vi "Set Frequency.vi"(8 "error in (no error)":errorcluster, 10 "Frequency (1000Hz)":dbl=1000.0, 11 "PWM in":refnum<class "LINX-PCA9865 PWM.lvclass">) -> (0 "error out":errorcluster, 3 "PWM out":refnum<class "LINX-PCA9865 PWM.lvclass">)   [LabVIEW 2019, in "LINX-PCA9865 PWM.lvclass"]
uses:
  LINX-PCA9865 PWM.lvclass
panel:
  out "Prescale Value":dbl
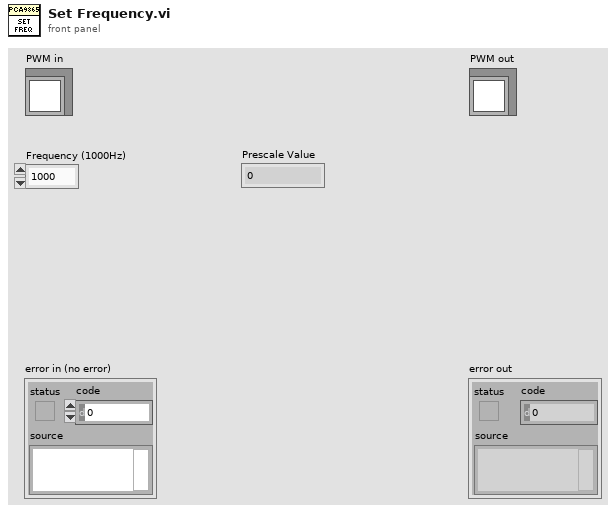
[diagram p1: front panel]
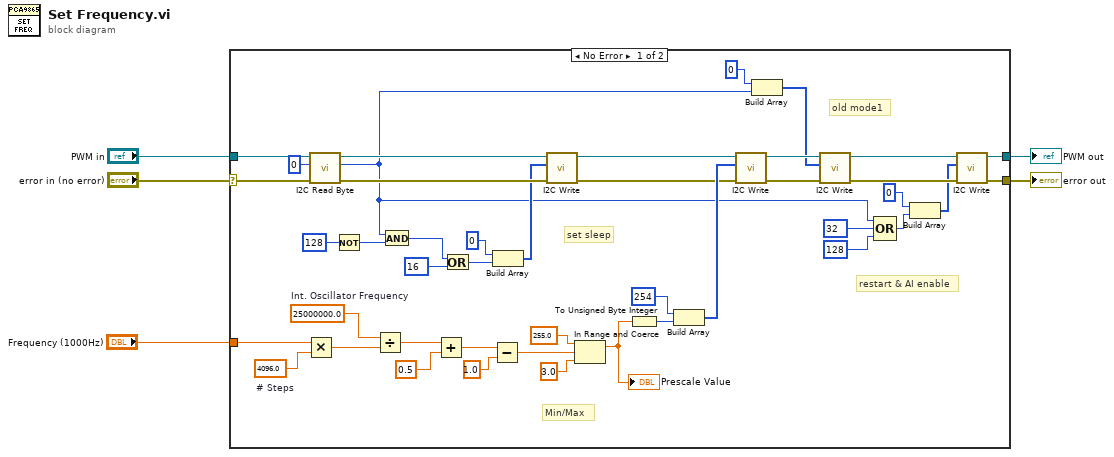
[diagram p0: block diagram]
diagram:
  n1 = case shown="No Error" "error in (no error)" {
    selector: "error in (no error)" -> [w32 w50]
    tunnel: [w13 w50] -> w4
    tunnel: [w12 w49] -> w2
    tunnel: "PWM in" -> [w33 w49]
    tunnel: "Frequency (1000Hz)" -> [w48 _]
    frame No Error {
      w47 = 4096.0  # # Steps
      w46 = 25000000.0  # Int. Oscillator Frequency
      # "set sleep"
      # "old mode1"
      # "restart & AI enable"
      # "Min/Max"
      n2 = Multiply(x=w48, y=w47) -> (x*y=w45:dbl)
      n3 = call "I2C Read Byte.vi"("error in (no error)"=w32, "Address"=u8 0, "LINX-PCA9865 PWM in"=w33) -> ("error out"=w26:errorcluster, "Byte Read"=w11:u8, "LINX-PCA9865 PWM out"=w23:refnum<class "LINX-PCA9865 PWM.lvclass">)  [unwired: 6 in]
      n4 = Not(x=u8 128) -> (.not. x?=w29:u8)
      n5 = Divide(x=w46, y=w45) -> (x/y=w44:dbl)
      n6 = And(x=w11, y=w29) -> (x .and. y?=w28:u8)
      n7 = Add(x=w44, y=0.5 ("x")) -> (x+y=w42:dbl)
      n8 = Or(x=w28, y=u8 16) -> (x .or. y?=w21:u8)
      n9 = Subtract(x=w42, y=1.0) -> (x-y=w40:dbl)
      n10 = Build Array(u8 0 ("Address"), w21) -> (w20:u8[])
      n11 = call "I2C Write.vi"("error in (no error)"=w26, "Bytes to Write"=w20, "LINX-PCA9865 PWM in"=w23) -> ("error out"=w25:errorcluster, "LINX-PCA9865 PWM out"=w24:refnum<class "LINX-PCA9865 PWM.lvclass">)  [unwired: 7 in]
      n12 = In Range and Coerce(upper limit=255.0, x=w40, lower limit=3.0) -> (coerced(x)=w37:dbl)  [unwired: 1 out]
      "Prescale Value" <- w37
      n13 = To Unsigned Byte Integer(number=w37) -> (unsigned 8bit integer=w36:u8)
      n14 = Build Array(u8 254 ("unsigned 8bit integer"), w36) -> (w35:u8[])
      n15 = call "I2C Write.vi"("error in (no error)"=w25, "Bytes to Write"=w35, "LINX-PCA9865 PWM in"=w24) -> ("error out"=w19:errorcluster, "LINX-PCA9865 PWM out"=w18:refnum<class "LINX-PCA9865 PWM.lvclass">)  [unwired: 7 in]
      n16 = Build Array(u8 0 ("Address"), w11) -> (w16:u8[])
      n17 = call "I2C Write.vi"("error in (no error)"=w19, "Bytes to Write"=w16, "LINX-PCA9865 PWM in"=w18) -> ("error out"=w14:errorcluster, "LINX-PCA9865 PWM out"=w15:refnum<class "LINX-PCA9865 PWM.lvclass">)  [unwired: 7 in]
      n18 = Compound Arithmetic op=OR(w11, u8 32, u8 128) -> (w7:u8)
      n19 = Build Array(u8 0 ("Address"), w7) -> (w6:u8[])
      n20 = call "I2C Write.vi"("error in (no error)"=w14, "Bytes to Write"=w6, "LINX-PCA9865 PWM in"=w15) -> ("error out"=w13:errorcluster, "LINX-PCA9865 PWM out"=w12:refnum<class "LINX-PCA9865 PWM.lvclass">)  [unwired: 7 in]
    }
    frame Error {
    }
  }
  "error out" <- w4
  "PWM out" <- w2
